vi "SCC Check In.vi"(6 "keep checked out? (F)":bool, 7 "advanced options":variant, 8 "error in (no error)":errorcluster, 9 "comment":string, 10 "files":path[](array[path]), 11 "source control reference in":T1) -> (0 "error out":errorcluster, 1 "dialog box cancelled?":bool, 2 "status message":string, 3 "source control reference out":T1)   [LabVIEW 2017, in "NI_SCC.lvlib"]
doc: "Checks in the specified files to source control."
uses:
  <vilib>/SourceControl/sccapi/NI_SCC.lvlib
  <vilib>/SourceControl/sccapi/SCCAPI Refnum.ctl
  <vilib>/SourceControl/sccapi/SCCAPI SCC Operations.ctl
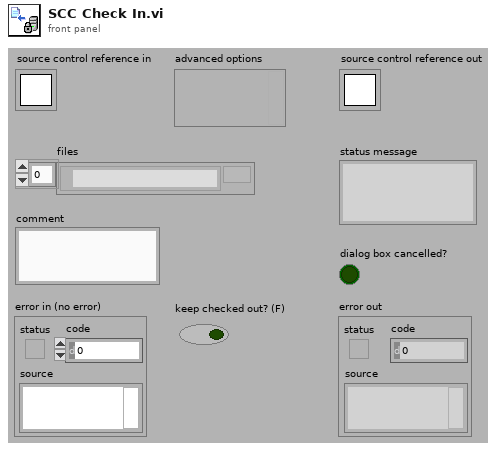
[diagram p1: front panel]
types:
  T1 = typedef "NI_SCC.lvlib/SCCAPI Refnum.ctl" = refnum<k1>
  T2 = typedef "NI_SCC.lvlib/SCCAPI SCC Operations.ctl" = enum16{"Add", "Check In", "Check Out", "Close Project", "Compare Files", "Compare VIs", "Configure Project", "File History", "File Properties", "File Status", "Find All Providers", "Get Advanced Command Options", "Get File Copy", "Get Latest Version", "Get Project Name", "Get StaticVI Path", "Initialize", "Not A Source Control Reference", "Open Project", "Provider Supports Functionality", "Remove", "Run Provider", "Undo Check Out", "Uninitialize", "Is File In Local Path"}
  T3 = typedef "SCCAPI Refnum.ctl" = refnum<k1>
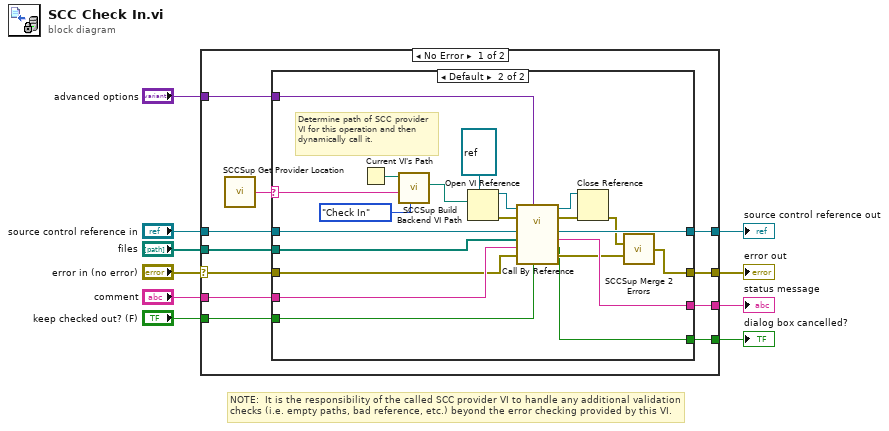
[diagram p0: block diagram]
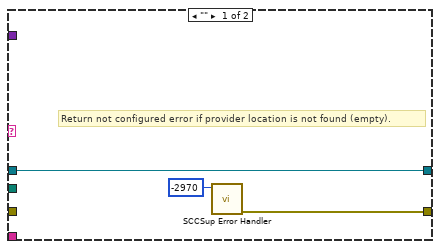
[diagram p2: hidden frame]
diagram:
  # "NOTE:  It is the responsibility of the called SCC provider VI to handle any additional validation checks (i.e. empty paths, bad reference, etc.) beyond the error checking provided by this VI."
  n1 = case shown="No Error" "error in (no error)" {
    selector: "error in (no error)" -> [w13 w47]
    tunnel: [w21 w47] -> w9
    tunnel: "source control reference in" -> [w20 w46]
    tunnel: [w19 _] -> w7
    tunnel: [w18 w46] -> w6
    tunnel: "files" -> [w17 _]
    tunnel: "comment" -> [w16 _]
    tunnel: "keep checked out? (F)" -> [w15 _]
    tunnel: [w12 _] -> w2
    tunnel: "advanced options" -> [w11 _]
    frame No Error {
      n2 = call <vilib>:"SCCSup Get Provider Location.vi"() -> ("provider location"=w14:string)  [unwired: 6 in]
      n3 = case shown="Default" w14 {
        selector: w14 -> [_ w28]
        tunnel: [w22 w45] -> w21
        tunnel: w20 -> [w24 w37]
        tunnel: [_ w44] -> w19
        tunnel: [w24 w38] -> w18
        tunnel: w17 -> [_ w36]
        tunnel: w16 -> [_ w35]
        tunnel: w15 -> [_ w34]
        tunnel: w13 -> [_ w27]
        tunnel: [_ w26] -> w12
        tunnel: w11 -> [_ w25]
        frame "" {
          # "Return not configured error if provider location is not found (empty)."
          n4 = call <vilib>:"SCCSup Error Handler.vi"("scc error code"=-2970 ("code")) -> ("error out"=w22:errorcluster)  [unwired: 10 in]
        }
        frame Default {
          # "Determine path of SCC provider VI for this operation and then dynamically call it."
          n5 = Current VI's Path() -> (path=w31:path)
          n6 = call <vilib>:"SCCSup Build Backend VI Path.vi"("scc operation"=SCCAPI_SCC_Operations."Check In", "provider location"=w28, "caller path"=w31) -> ("scc backend VI path"=w30:path)  [unwired: 8 in]
          n7 = Open VI Reference(type specifier VI Refnum (for type only)=refnum<vi> refnum, vi path=w30) -> (vi reference=w42:refnum<vi>, error out=w41:errorcluster)  [unwired: 4 in]
          n8 = call-by-ref "?"(reference=w42, error in=w41, "keep checked out? (F)"=w34, "advanced options"=w25, "error in (no error)"=w27, "comment"=w35, "files"=w36, "source control reference in"=w37) -> (reference out=w40:refnum<vi>, error out=w39:errorcluster, 0:"error out"=w32:errorcluster, "dialog box cancelled?"=w26:bool, "status message"=w44:string, "source control reference out"=w38:T3)  [unwired: 2 in]
          n9 = Close Reference(reference=w40, error in (no error)=w39) -> (error out=w33:errorcluster)
          n10 = call <vilib>:"SCCSup Merge 2 Errors.vi"("Error IO 1"=w33, "Error IO 2"=w32) -> ("Error IO out"=w45:errorcluster)  [unwired: 13 in]
        }
      }
    }
    frame Error {
    }
  }
  "error out" <- w9
  "status message" <- w7
  "source control reference out" <- w6
  "dialog box cancelled?" <- w2
